vi "Read dRA.vi"(8 "error in (no error)":errorcluster, 11 "DifftrackStatus in":refnum<class "DifftrackStatus.lvclass">) -> (0 "error out":errorcluster, 2 "dRA_ArcsPS":dbl[unit] min=0.0 max=4.84813681109536e-05, 3 "DifftrackStatus out":refnum<class "DifftrackStatus.lvclass">)   [LabVIEW 2014, in "TCSDataDefinitions.lvlib" / "TCSPublicStatus.lvlib" / "PointingPositions.lvlib" / "DifftrackStatus.lvclass"]
uses:
  DifftrackStatus.lvclass
  DifftrackStatus.lvclass/DifftrackStatus.ctl
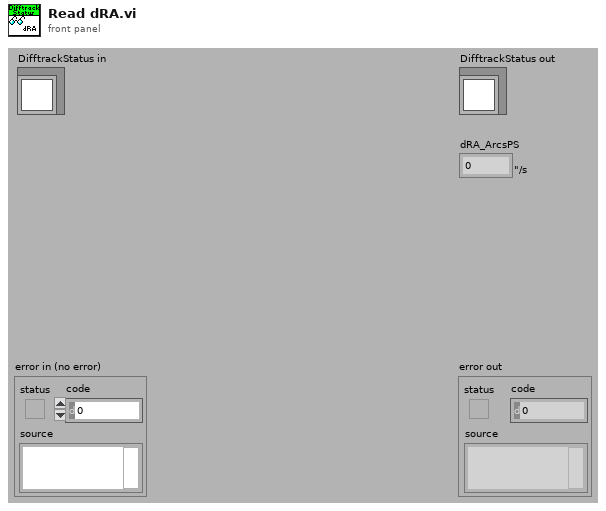
[diagram p1: front panel]
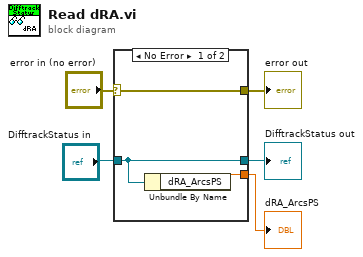
[diagram p0: block diagram]
diagram:
  n1 = case shown="No Error" "error in (no error)" {
    selector: "error in (no error)" -> [w8 w9]
    tunnel: [w8 w9] -> w4
    tunnel: [w7 w10] -> w2
    tunnel: "DifftrackStatus in" -> [w7 w10]
    tunnel: [w6 _] -> w1
    frame No Error {
      n2 = Unbundle By Name(w7) -> ("dRA_ArcsPS"=w6:dbl[unit])
    }
    frame Error {
    }
  }
  "error out" <- w4
  "dRA_ArcsPS" <- w1
  "DifftrackStatus out" <- w2
